vi "Populate Tree.vi"(10 "Tree In":refnum<vi>, 11 "Tree":T1[](array[typedef])) -> ()   [LabVIEW 2020, in "Linker Info.lvlib"]
uses:
  Linker Info.lvlib
  Tree Item.ctl
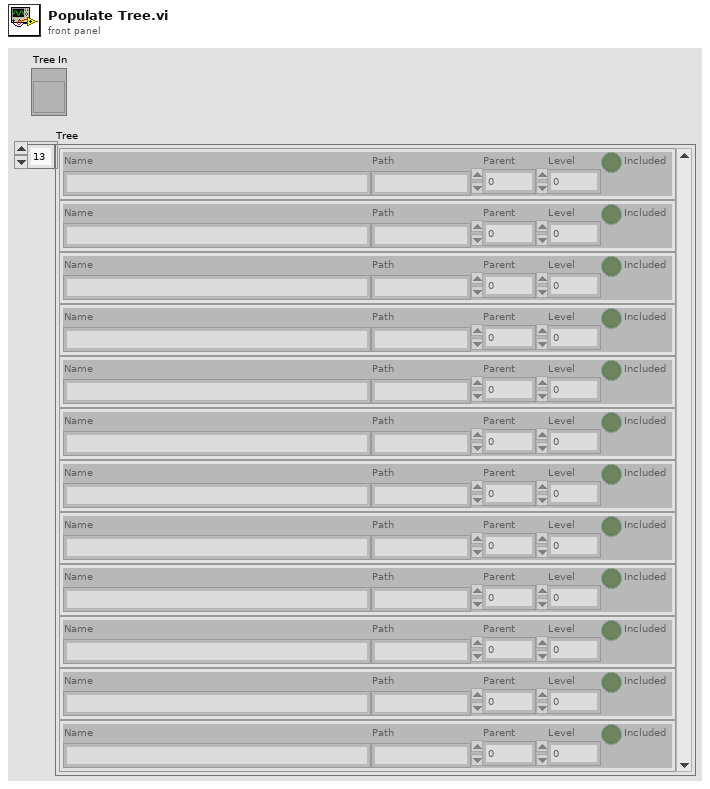
[diagram p1: front panel]
types:
  T1 = typedef "Linker Info.lvlib/Tree Item.ctl" = cluster{"Name":string, "Path":string, "Parent":i32, "Level":i32, "Included":bool}
  T2 = cluster{"Left Cell String":string, "Child Text":string[], "Child Tag":string, "Item Indent":i32, "Child Only?":bool, "Glyph Index":i32}
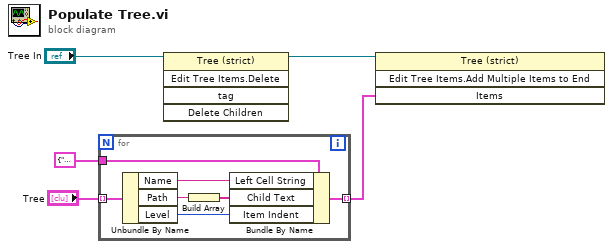
[diagram p0: block diagram]
diagram:
  n1 = for {
    tunnel: "Tree" -> [w12] mode=indexing
    tunnel: T2 {"Left Cell String"="", "Child Text"=[], "Child Tag"="", "Item Indent"=0, "Child Only?"=FALSE, "Glyph Index"=0} ("Item") -> [w11]
    tunnel: [w6] -> w1 mode=indexing
    n2 = Unbundle By Name(w12) -> ("Name"=w10:string, "Path"=w9:string, "Level"=w7:i32)
    n3 = Build Array(w9) -> (w8:string[])
    n4 = Bundle By Name(cluster=w11, "Left Cell String"=w10, "Child Text"=w8, "Item Indent"=w7) -> (w6:T2)
  }
  n5 = invoke class="Tree (strict)" method="Edit Tree Items.Delete"(reference="Tree In") -> (reference out=w4:refnum<vi>)  [unwired: 4 in, 4 out]
  n6 = invoke class="Tree (strict)" method="Edit Tree Items.Add Multiple Items to End"(reference=w4, "Items"=w1) -> ()  [unwired: 2 in, 4 out]
